vi "test_open.vi"() -> ()   [LabVIEW 2018]
panel:
  in  "ICImagingControl":refnum<k7>(container)
  out "Devices":string[](array[string])
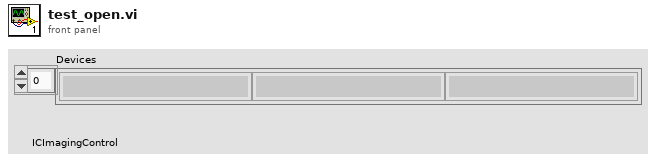
[diagram p1: front panel]
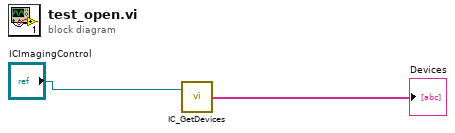
[diagram p0: block diagram]
diagram:
  n1 = call <userlib>:"IC_GetDevices.vi"("ICImagingControl In"="ICImagingControl") -> ("Devices"=→"Devices":string[])  [unwired: 1 in, 2 out]
